vi "ZeroDriveSpeed.vi"(8 "error in (no error)":errorcluster) -> (0 "error out":errorcluster)   [LabVIEW 2016, in "DriveBase.lvclass"]
uses:
  DriveBase.lvclass
  DriveStates.ctl
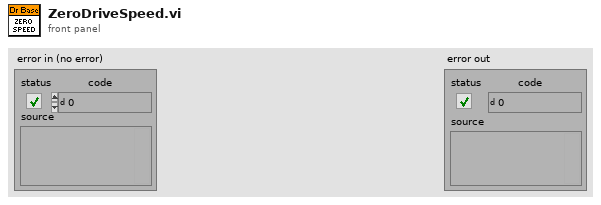
[diagram p1: front panel]
types:
  T1 = typedef "DriveBase.lvclass/DriveStates.ctl" = enum16{"Tank", "Arcade", "DriveStraight"}
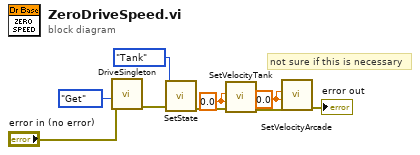
[diagram p0: block diagram]
diagram:
  w3 = 0.0 ("Y Axis")
  w5 = 0.0 ("leftVelocitySetpointInput")
  # "not sure if this is necessary"
  n1 = call "DriveSingleton.vi"("error in (no error)"="error in (no error)", "Get/Set"=enum16{"Get", "Set"}."Get") -> ("error out"=w8:errorcluster)  [unwired: 8 in, 1 out]
  n2 = call "SetState.vi"("error in (no error)"=w8, "State"=DriveStates."Tank") -> ("error out"=w6:errorcluster)  [unwired: 9 in]
  n3 = call "SetVelocityTank.vi"("error in (no error)"=w6, "leftVelocitySetpointInput"=w5, "rightVelocitySetpointInput"=w5) -> ("error out"=w4:errorcluster)  [unwired: 8 in]
  n4 = call "SetVelocityArcade.vi"("error in (no error)"=w4, "Y Axis"=w3, "X Axis"=w3) -> ("error out"=→"error out":errorcluster)  [unwired: 8 in]
